vi "Get Table Rows by Column Value (VAR).vi"(6 "Column Value":variant, 7 "Sheet Name":string, 8 "error in":errorcluster, 9 "Column Name":string, 10 "Table Name":string, 11 "SpreadsheetDoc in":refnum<k24>) -> (0 "error out":errorcluster, 2 "Cell Values":variant[][](array[variant]), 3 "SpreadsheetDoc out":refnum<k24>)   [LabVIEW 2019, in "Open Xml.lvlib"]
uses:
  Open Xml.lvlib
  D:/git/Open-Xml-LabVIEW/Source/DocumentFormat.OpenXml.dll
  DocumentFormat.OpenXml.dll
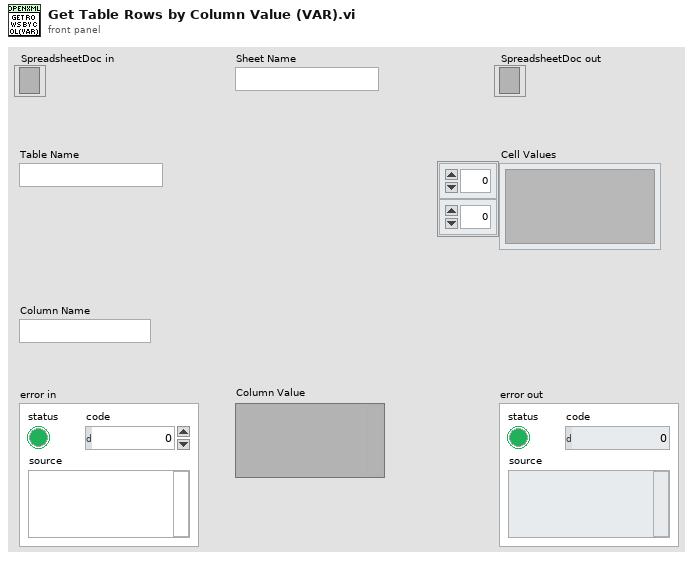
[diagram p1: front panel]
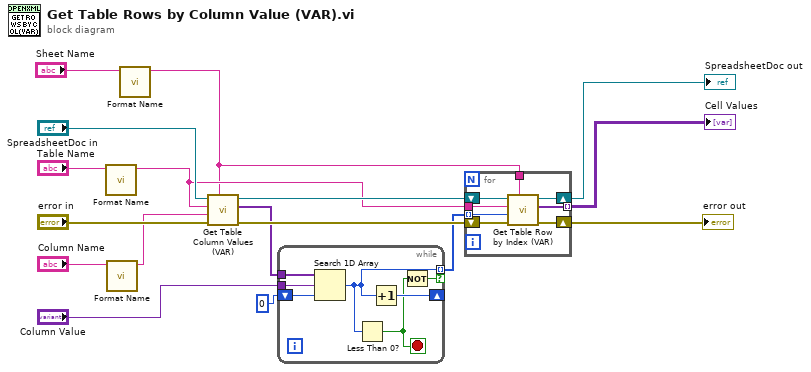
[diagram p0: block diagram]
diagram:
  n1 = call "Format Name.vi"("Sheet Name"="Table Name") -> ("Formatted Sheet Name"=w3:string)  [unwired: 10 in]
  n2 = call "Format Name.vi"("Sheet Name"="Column Name") -> ("Formatted Sheet Name"=w1:string)  [unwired: 10 in]
  n3 = call "Format Name.vi"("Sheet Name"="Sheet Name") -> ("Formatted Sheet Name"=w2:string)  [unwired: 10 in]
  n4 = call "Get Table Column Values (VAR).vi"("Sheet Name in"=w2, "error in"="error in", "Column Name"=w1, "Table Name"=w3, "SpreadsheetDoc in"="SpreadsheetDoc in") -> ("error out"=w12:errorcluster, "Column Values"=w9:variant[], "SpreadsheetDoc out"=w11:refnum<k24>)  [unwired: 4 in]
  n5 = while {
    tunnel: w9 -> [w24]
    tunnel: "Column Value" -> [w23]
    shift-right: [w21] -> _
    shift-left: 0 -> [w22]
    tunnel: [w20] -> w4 mode=indexing if=w18
    stop <- w19 stop-if-true
    n6 = Search 1D Array(1D array=w24, element=w23, start index (0)=w22) -> (index of element=w20:i32)
    n7 = Less Than 0?(x=w20) -> (x < 0?=w19:bool)
    n8 = Increment(x=w20) -> (x+1=w21:i32)
    n9 = Not(x=w19) -> (.not. x?=w18:bool)
  }
  n10 = for {
    tunnel: [w30] -> w15 mode=indexing
    tunnel: w2 -> [w27]
    tunnel: w3 -> [w26]
    tunnel: w4 -> [w25] mode=indexing
    shift-right: [w32] -> w17
    shift-left: w12 -> [w29]
    shift-right: [w31] -> w16
    shift-left: w11 -> [w28]
    n11 = call "Get Table Row by Index (VAR).vi"("Sheet Name"=w27, "error in"=w29, "Row Index"=w25, "Table Name"=w26, "SpreadsheetDoc in"=w28) -> ("error out"=w32:errorcluster, "Rows"=w30:variant[], "SpreadsheetDoc out"=w31:refnum<k24>)  [unwired: 4 in]
  }
  "SpreadsheetDoc out" <- w16
  "error out" <- w17
  "Cell Values" <- w15
